vi "20211015_06.vi"() -> ()   [LabVIEW 2019]
panel:
  out "已婚":bool
  out "年齡":i32
  out "姓名":string
  in  "個人資料":cluster{"姓名":string, "年齡":i32, "已婚":bool}={"姓名"="吳幗彰", "年齡"=80, "已婚"=FALSE}
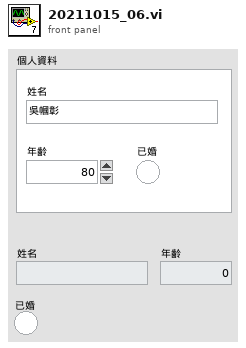
[diagram p1: front panel]
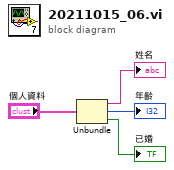
[diagram p0: block diagram]
diagram:
  n1 = Unbundle("個人資料") -> ("姓名"=→"姓名":string, "年齡"=→"年齡":i32, "已婚"=→"已婚":bool)
